vi "ti2_setHome.vi"(8 "error in (no error)":errorcluster) -> (0 "error out":errorcluster)   [LabVIEW 2018, in "ti2lv.lvlib"]
uses:
  ti2lv.lvlib
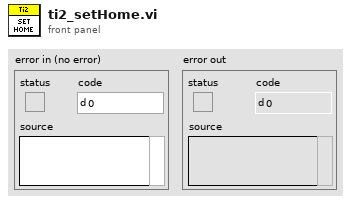
[diagram p1: front panel]
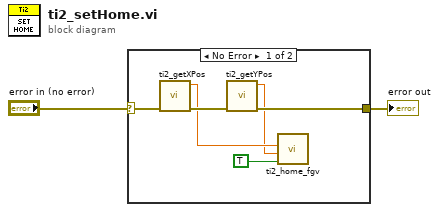
[diagram p0: block diagram]
diagram:
  n1 = case shown="No Error" "error in (no error)" {
    selector: "error in (no error)" -> [w8 w9]
    tunnel: [w6 w9] -> w2
    frame No Error {
      n2 = call "ti2_getXPos.vi"("error in (no error)"=w8) -> ("error out"=w7:errorcluster, "x Position (um)"=w5:dbl)  [unwired: 9 in]
      n3 = call "ti2_getYPos.vi"("error in (no error)"=w7) -> ("error out"=w6:errorcluster, "y Position (um)"=w4:dbl)  [unwired: 9 in]
      n4 = call "ti2_home_fgv.vi"("Init?"=TRUE, "Y Init  (um)"=w4, "X Init (um)"=w5) -> ()  [unwired: 7 in, 2 out]
    }
    frame Error {
    }
  }
  "error out" <- w2
